vi "Take Picture Flir-Ax8.vi"(1 "Take Picture":bool, 2 "Image":T1) -> (0 "Reset Button":bool)   [LabVIEW 2016]
uses:
  <vilib>/vision/Image Controls.llb/IMAQ Image.ctl
  Global Flir-Ax8.vi
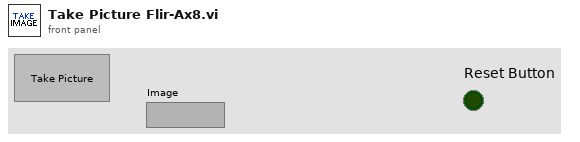
[diagram p1: front panel]
types:
  T1 = typedef "IMAQ Image.ctl" = refnum<image>
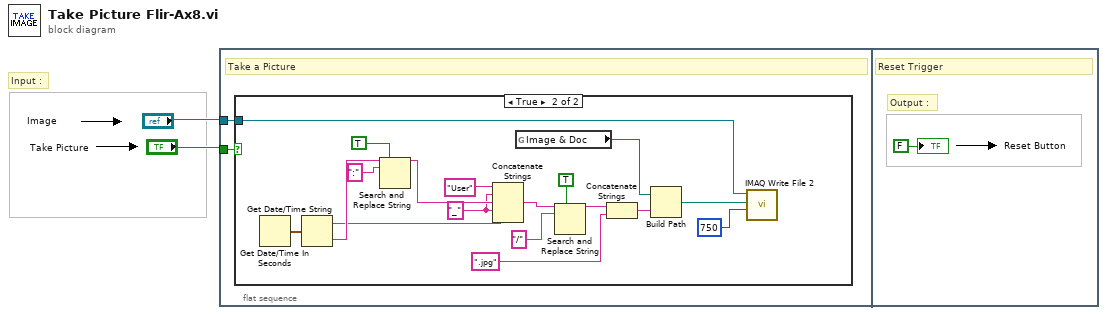
[diagram p0: block diagram]
diagram:
  # "Input :"
  n1 = flat-sequence {
    tunnel: "Take Picture" -> [w4]
    tunnel: "Image" -> [w3]
    frame #0 {
      # "Take a Picture"
      n2 = case shown="True" w4 {
        tunnel: w3 -> [_ w6]
        frame False {
        }
        frame True {
          w10 = "_" ("string")
          n3 = Get Date/Time In Seconds() -> (seconds since 1Jan1904=w19:timestamp)
          n4 = Get Date/Time String(seconds (now)=w19) -> (date string=w14:string, time string=w16:string)  [unwired: 2 in]
          n5 = Search and Replace String(replace all?=TRUE ("replace all? (F)"), input string=w16, search string=":") -> (result string=w15:string)  [unwired: 5 in, 3 out]
          n6 = Concatenate Strings ("add")("User" ("string"), w10, w15, w10, w14) -> (w13:string)
          n7 = global read "Global Flir-Ax8.vi" "Image & Doc"() -> (w5:path)
          n8 = Search and Replace String(replace all?=TRUE ("replace all? (F)"), input string=w13, search string="/") -> (result string=w12:string)  [unwired: 5 in, 3 out]
          n9 = Concatenate Strings ("add")(w12, ".jpg" ("string")) -> (w22:string)
          n10 = Build Path(base path=w5, name or relative path=w22) -> (appended path=w8:path)
          n11 = call-poly "IMAQ Write File 2"("Image Quality"=u32 750, "File Path"=w8, "Image"=w6) -> ()  [unwired: 7 in, 2 out]
        }
      }
    }
    frame #1 {
      # "Output :"
      # "Reset Trigger"
      "Reset Button" <- FALSE ("Boolean")
    }
  }
